vi "Tipper-Solenoids.vi"(1 "Deploy Tipper":bool) -> (0 "Tipper Locked":bool)   [LabVIEW 2011]
uses:
  Robot Global Data.vi
  <vilib>/Rock Robotics/WPI/Solenoid/Deprecated/WPI_SolenoidSetBool.vi
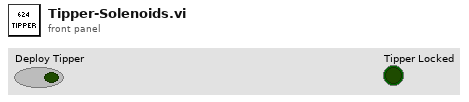
[diagram p1: front panel]
types:
  T1 = typedef "WPI_SolenoidDevRef.ctl" = cluster{"DevStatus":errorcluster, "Solenoid Module":T2, "Forward Solenoid Channel":T3, "Reverse Solenoid Channel":T3}
  T2 = typedef "FPGA_TypedefSolenoidModule.ctl" = enum16{"Solenoid Module 1", "Solenoid Module 2"}
  T3 = typedef "WPI_SolenoidChannel.ctl" = enum8{"Solenoid 1", "Solenoid 2", "Solenoid 3", "Solenoid 4", "Solenoid 5", "Solenoid 6", "Solenoid 7", "Solenoid 8", "Invalid"}
  T4 = typedef "WPI_DigitalInputDevRef.ctl" = cluster{"DevStatus":errorcluster, "DIO Channel":T5, "Digital Module":T6}
  T5 = typedef "FPGA_DIOChannel.ctl" = enum8{"DIO 1", "DIO 2", "DIO 3", "DIO 4", "DIO 5", "DIO 6", "DIO 7", "DIO 8", "DIO 9", "DIO 10", "DIO 11", "DIO 12", "DIO 13", "DIO 14", "Invalid"}
  T6 = typedef "FPGA_TypedefDigitalModule.ctl" = enum16{"Digital Module 1", "Digital Module 2"}
  T7 = cluster{"Gear Shifter":bool, "Tipper":bool, "Tipper Lock":bool, "Stabilizer":bool}
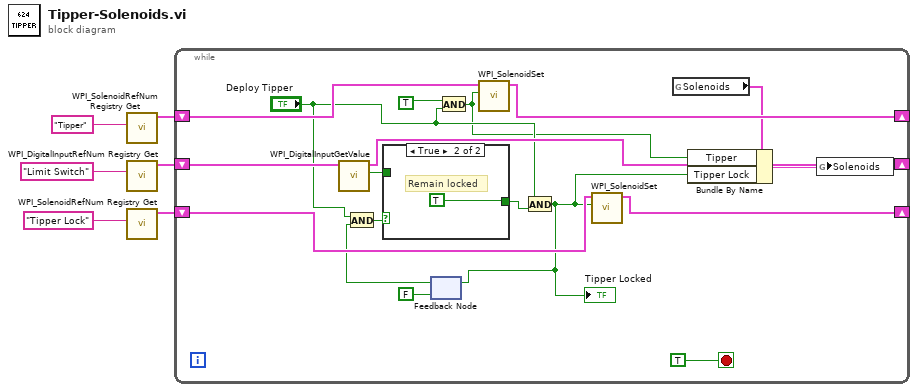
[diagram p0: block diagram]
diagram:
  n1 = call <vilib>:"WPI_SolenoidRefNum Registry Get.vi"("refnum name"="Tipper") -> ("SolenoidDevRef"=w1:T1)  [unwired: 9 in, 1 out]
  n2 = call <vilib>:"WPI_DigitalInputRefNum Registry Get.vi"("refnum name"="Limit Switch") -> ("DigitalInputDevRef"=w2:T4)  [unwired: 9 in, 1 out]
  n3 = call <vilib>:"WPI_SolenoidRefNum Registry Get.vi"("refnum name"="Tipper Lock") -> ("SolenoidDevRef"=w3:T1)  [unwired: 9 in, 1 out]
  n4 = while {
    shift-right: [w22] -> _
    shift-left: w3 -> [w23]
    shift-right: [w20] -> _
    shift-left: w2 -> [w21]
    shift-right: [w18] -> _
    shift-left: w1 -> [w19]
    stop <- TRUE stop-if-true
    n5 = call <vilib>:"WPI_DigitalInputGetValue.vi"("DigitalInputDevRef"=w21) -> ("Value"=w15:bool, "DigitalInputDevRef"=w20:T4)  [unwired: 8 in, 1 out]
    n6 = feedback #1(FALSE ("Value")) -> (w12:bool)
    n7 = And(x="Deploy Tipper", y=w12) -> (x .and. y?=w13:bool)
    n8 = case shown="True" w13 {
      tunnel: [w25 TRUE] -> w16
      tunnel: w15 -> [w25 _]
      frame False {
      }
      frame True {
        # "Remain locked"
      }
    }
    n9 = And(x=TRUE, y="Deploy Tipper") -> (x .and. y?=w7:bool)
    n10 = call-poly <vilib>:"WPI_SolenoidSet.vi"("Value"=w7, "SolenoidDevRef"=w19) -> ("SolenoidDevRef"=w18:T1)  [unwired: 8 in, 1 out]
    n11 = And(x="Deploy Tipper", y=w16) -> (x .and. y?=w8:bool)
    "Tipper Locked" <- w8
    n12 = feedback-in #1(w8) -> ()
    n13 = call-poly <vilib>:"WPI_SolenoidSet.vi"("Value"=w8, "SolenoidDevRef"=w23) -> ("SolenoidDevRef"=w22:T1)  [unwired: 8 in, 1 out]
    n14 = global read "Robot Global Data.vi" "Solenoids"() -> (w9:T7)
    n15 = Bundle By Name(cluster=w9, "Tipper"=w7, "Tipper Lock"=w8) -> (w10:T7)
    n16 = global write "Robot Global Data.vi" "Solenoids"(w10) -> ()
  }
